vi "Read Buses.vi"(8 "error in (no error)":errorcluster, 11 "Fault-Injection Bus in":refnum<class "Fault-Injection Bus.lvclass">) -> (0 "error out":errorcluster, 2 "Buses":refnum<class "Bus_Access.lvclass">[](array[class]), 3 "Fault-Injection Bus out":refnum<class "Fault-Injection Bus.lvclass">)   [LabVIEW 2021, in "Fault-Injection Bus.lvclass"]
uses:
  Fault-Injection Bus.lvclass
  Fault-Injection Bus.lvclass/Fault-Injection Bus.ctl
  Omni-Bus/Bus Access/Bus_Access.lvclass
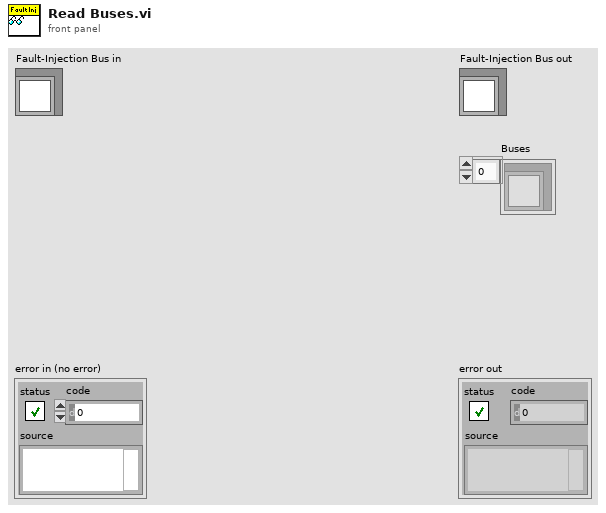
[diagram p1: front panel]
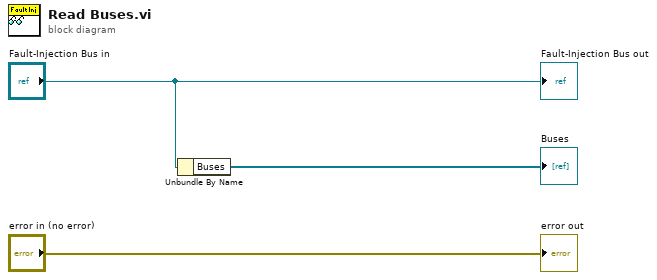
[diagram p0: block diagram]
diagram:
  n1 = Unbundle By Name("Fault-Injection Bus in") -> ("Buses"=→"Buses":refnum<class "Bus_Access.lvclass">[])
  "error out" <- "error in (no error)"
  "Fault-Injection Bus out" <- "Fault-Injection Bus in"
